vi "C,D,E Value Change.vi"(9 "E":T2 {"Y2" scale=0.0..10.0; "Y1" scale=0.0..10.0; "X2" scale=0.0..10.0; "X1" scale=0.0..10.0}, 10 "D":T2 {"Y2" scale=0.0..10.0; "Y1" scale=0.0..10.0; "X2" scale=0.0..10.0; "X1" scale=0.0..10.0}, 11 "C":T2 {"Y2" scale=0.0..10.0; "Y1" scale=0.0..10.0; "X2" scale=0.0..10.0; "X1" scale=0.0..10.0}) -> (0 "C,D,E Cluster":T1, 1 "E":T2, 2 "D":T2, 3 "C":T2)   [LabVIEW 2017]
uses:
  Acquisition/Typedefs/nonlinearRamps_CDE.ctl
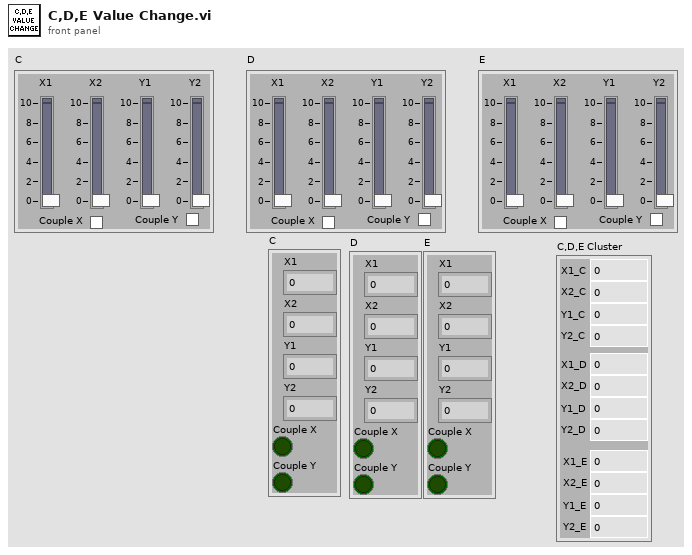
[diagram p1: front panel]
types:
  T1 = typedef "nonlinearRamps_CDE.ctl" = cluster{"X1_C":dbl, "X2_C":dbl, "Y1_C":dbl, "Y2_C":dbl, "X1_D":dbl, "X2_D":dbl, "Y1_D":dbl, "Y2_D":dbl, "X1_E":dbl, "X2_E":dbl, "Y1_E":dbl, "Y2_E":dbl}
  T2 = cluster{"X1":dbl, "X2":dbl, "Y1":dbl, "Y2":dbl, "Couple X":bool, "Couple Y":bool}
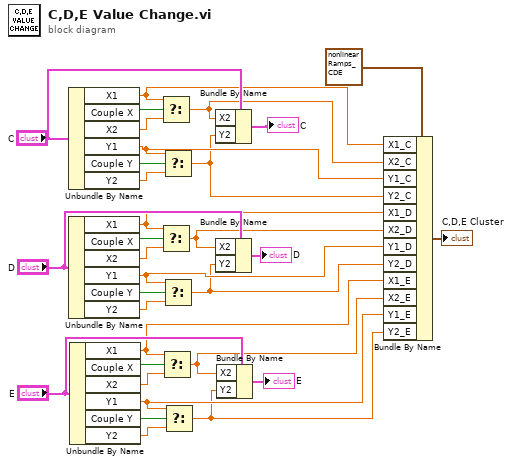
[diagram p0: block diagram]
diagram:
  n1 = Unbundle By Name("C") -> ("X1"=w13:dbl, "Couple X"=w32:bool, "X2"=w31:dbl, "Y1"=w11:dbl, "Couple Y"=w30:bool, "Y2"=w29:dbl)
  n2 = Unbundle By Name("D") -> ("X1"=w9:dbl, "Couple X"=w24:bool, "X2"=w25:dbl, "Y1"=w7:dbl, "Couple Y"=w26:bool, "Y2"=w27:dbl)
  n3 = Unbundle By Name("E") -> ("X1"=w5:dbl, "Couple X"=w23:bool, "X2"=w22:dbl, "Y1"=w3:dbl, "Couple Y"=w21:bool, "Y2"=w20:dbl)
  n4 = Select(t=w13, s=w32, f=w31) -> (s? t:f=w12:dbl)
  n5 = Select(t=w9, s=w24, f=w25) -> (s? t:f=w8:dbl)
  n6 = Select(t=w5, s=w23, f=w22) -> (s? t:f=w4:dbl)
  n7 = Select(t=w11, s=w30, f=w29) -> (s? t:f=w10:dbl)
  n8 = Select(t=w7, s=w26, f=w27) -> (s? t:f=w6:dbl)
  n9 = Select(t=w3, s=w21, f=w20) -> (s? t:f=w2:dbl)
  n10 = Bundle By Name(cluster="C", "X2"=w12, "Y2"=w10) -> (→"C":T2)
  n11 = Bundle By Name(cluster="D", "X2"=w8, "Y2"=w6) -> (→"D":T2)
  n12 = Bundle By Name(cluster="E", "X2"=w4, "Y2"=w2) -> (→"E":T2)
  n13 = Bundle By Name(cluster=T1 {"X1_C"=0.0, "X2_C"=0.0, "Y1_C"=0.0, "Y2_C"=0.0, "X1_D"=0.0, "X2_D"=0.0, "Y1_D"=0.0, "Y2_D"=0.0, "X1_E"=0.0, "X2_E"=0.0, "Y1_E"=0.0, "Y2_E"=0.0} ("C,D,E Parameters In"), "X1_C"=w13, "X2_C"=w12, "Y1_C"=w11, "Y2_C"=w10, "X1_D"=w9, "X2_D"=w8, "Y1_D"=w7, "Y2_D"=w6, "X1_E"=w5, "X2_E"=w4, "Y1_E"=w3, "Y2_E"=w2) -> (→"C,D,E Cluster":T1)
